vi "Get Parameter Bit Encoding.vi"(8 "error in":errorcluster, 11 "parameter ref in":T2 format="%.0x") -> (0 "error out":errorcluster, 1 "number of bits":i32, 2 "start bit":i32, 3 "parameter ref out":T2 format="%.0x", 5 "signed?":bool, 7 "encoding type":T1)   [LabVIEW 2020, in "ARINC 429 Scripting.lvlib"]
uses:
  ARINC 429 Scripting.lvlib
  <vilib>/NI VeriStand/Custom Device API/Custom Device Item Ref.ctl
  Encoding and Decoding/Encoding.ctl
  Ballard/Constants.vi
  <vilib>/NI VeriStand/Custom Device API/Get Item Property (U16).vi
  <vilib>/NI VeriStand/Custom Device API/Get Item Property (I32).vi
  <vilib>/NI VeriStand/Custom Device API/Get Item Property (Boolean).vi
  <vilib>/NI VeriStand/Custom Device API/Custom Device API.lvlib
  Ballard/Ballard ARINC 429 Scripting.lvlib
  Encoding and Decoding/Encoding and Decoding.lvlib
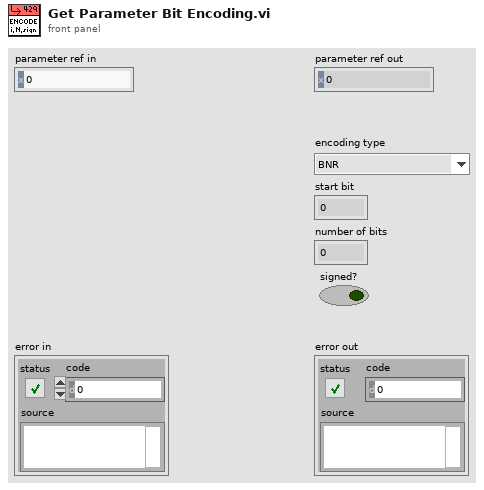
[diagram p1: front panel]
types:
  T1 = typedef "Encoding and Decoding.lvlib/Encoding.ctl" = enum16{"BNR", "BCD", "Discrete"}
  T2 = typedef "Custom Device API.lvlib/Custom Device Item Ref.ctl" = u64
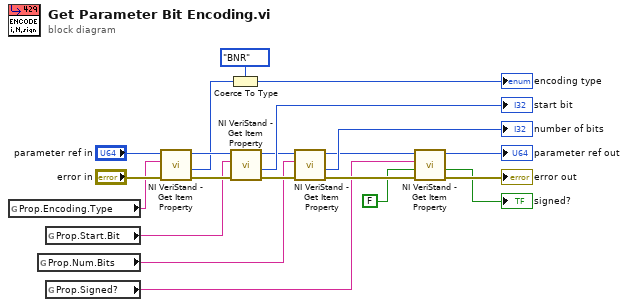
[diagram p0: block diagram]
diagram:
  n1 = global read "Constants.vi" "Prop.Encoding.Type"() -> (w6:string)
  n2 = global read "Constants.vi" "Prop.Num.Bits"() -> (w4:string)
  n3 = global read "Constants.vi" "Prop.Start.Bit"() -> (w5:string)
  n4 = global read "Constants.vi" "Prop.Signed?"() -> (w8:string)
  n5 = call-poly <vilib>:"NI VeriStand - Get Item Property.vi"("error in (no error)"="error in", "Property Name"=w6, "Item Ref in"="parameter ref in") -> ("error out"=w13:errorcluster, "Value"=w2:u16, "Item Ref out"=w14:T2)  [unwired: 5 in, 1 out]
  n6 = Coerce To Type(0:w2, 1:Encoding."BNR" ("encoding type")) -> (2:→"encoding type":T1)
  n7 = call-poly <vilib>:"NI VeriStand - Get Item Property.vi"("error in (no error)"=w13, "Property Name"=w5, "Item Ref in"=w14) -> ("error out"=w11:errorcluster, "Value"=→"start bit":i32, "Item Ref out"=w12:T2)  [unwired: 5 in, 1 out]
  n8 = call-poly <vilib>:"NI VeriStand - Get Item Property.vi"("error in (no error)"=w11, "Property Name"=w4, "Item Ref in"=w12) -> ("error out"=w9:errorcluster, "Value"=→"number of bits":i32, "Item Ref out"=w10:T2)  [unwired: 5 in, 1 out]
  n9 = call-poly <vilib>:"NI VeriStand - Get Item Property.vi"("error in (no error)"=w9, "Default Value"=FALSE, "Property Name"=w8, "Item Ref in"=w10) -> ("error out"=→"error out":errorcluster, "Value"=→"signed?":bool, "Item Ref out"=→"parameter ref out":T2)  [unwired: 4 in, 1 out]
